vi "Equip-Get Active Sources.vi"(0 "error in":errorcluster, 7 "Source Names":string[](array[string])) -> (4 "error out":errorcluster, 10 "Names":string[](array[string]), 15 "Chans":i32[](array[numeric]))   [LabVIEW 2020]
uses:
  <vilib>/Utility/config.llb/Read Key (String).vi
  <vilib>/Utility/config.llb/Read Key (I32).vi
  <vilib>/Utility/config.llb/NI_LVConfig.lvlib
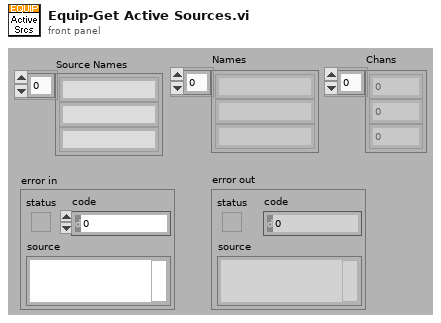
[diagram p1: front panel]
types:
  T1 = typedef "NI_LVConfig.lvlib/Config Data RefNum.ctl" = refnum<k1>
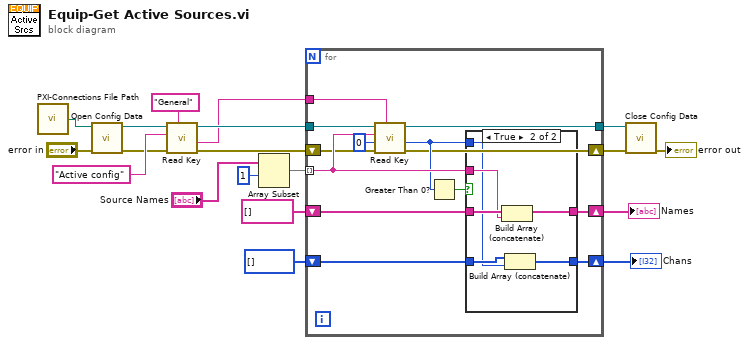
[diagram p0: block diagram]
diagram:
  n1 = call "PXI-Connections File Path.vi"() -> ("Path"=w1:path)  [unwired: 1 in]
  n2 = call <vilib>:"Open Config Data.vi"("error in (no error)"="error in", "configuration file path"=w1) -> ("error out"=w10:errorcluster, "refnum"=w11:T1)  [unwired: 7 in, 1 out]
  n3 = call-poly <vilib>:"Read Key.vi"("section"="General", "error in (no error)"=w10, "key"="Active config" ("section"), "refnum"=w11) -> ("error out"=w8:errorcluster, "value"=w6:string, "refnum out"=w7:T1)  [unwired: 4 in, 1 out]
  n4 = Array Subset(array="Source Names", index=1) -> (w18:string[])  [unwired: 1 in]
  n5 = for {
    tunnel: w18 -> [w29] mode=indexing
    tunnel: w7 -> [w32]
    tunnel: w6 -> [w20]
    shift-right: [w26] -> w15
    shift-left: string[] [] ("AO Names") -> [w27]
    shift-right: [w24] -> w14
    shift-left: i32[] [] ("AI Chans") -> [w25]
    shift-right: [w23] -> w4
    shift-left: w8 -> [w22]
    tunnel: [w21] -> w3
    n6 = call-poly <vilib>:"Read Key.vi"("section"=w20, "error in (no error)"=w22, "default value"=0, "key"=w29, "refnum"=w32) -> ("error out"=w23:errorcluster, "value"=w28:i32, "refnum out"=w21:T1)  [unwired: 3 in, 1 out]
    n7 = Greater Than 0?(x=w28) -> (x > 0?=w30:bool)
    n8 = case shown="True" w30 {
      tunnel: w29 -> [_ w38]
      tunnel: w28 -> [_ w35]
      tunnel: w27 -> [w34 w39]
      tunnel: [w34 w40] -> w26
      tunnel: w25 -> [w33 w36]
      tunnel: [w33 w37] -> w24
      frame False {
      }
      frame True {
        n9 = Build Array (concatenate)(w39, w38) -> (w40:string[])
        n10 = Build Array (concatenate)(w36, w35) -> (w37:i32[])
      }
    }
  }
  "Names" <- w15
  "Chans" <- w14
  n11 = call <vilib>:"Close Config Data.vi"("error in (no error)"=w4, "refnum"=w3) -> ("error out"=→"error out":errorcluster)  [unwired: 8 in, 1 out]
